vi "CreateXnYVector.vi"(8 "Line Count":i32, 9 "Pixel Count":i32, 10 "Y Step Size":dbl, 11 "X Step Size":dbl) -> (2 "Array 2":dbl[](array[numeric]), 3 "Array":dbl[](array[numeric]))   [LabVIEW 2020]
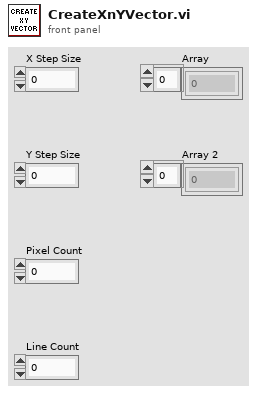
[diagram p1: front panel]
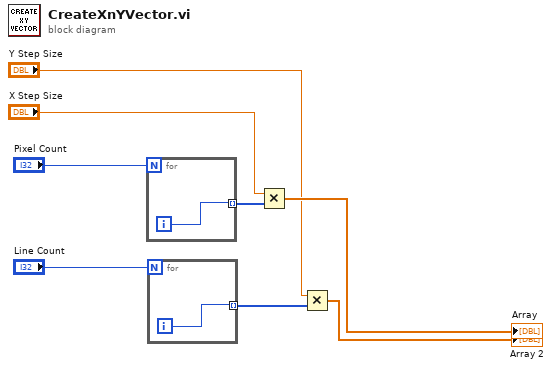
[diagram p0: block diagram]
diagram:
  n1 = for {
    N: "Pixel Count" -> [_]
    tunnel: [w9] -> w3 mode=indexing
    i -> [w9]
  }
  n2 = for {
    N: "Line Count" -> [_]
    tunnel: [w10] -> w5 mode=indexing
    i -> [w10]
  }
  n3 = Multiply(x="X Step Size", y=w3) -> (x*y=→"Array":dbl[])
  n4 = Multiply(x="Y Step Size", y=w5) -> (x*y=→"Array 2":dbl[])
